vi "Start Daq.vi"(4 "AI voltage":dbl[](array[numeric]), 6 "AI Channels":string[](array[string]), 8 "error in":errorcluster, 9 "samples per read":i32=10 min=1 step=1, 10 "Data rate (hz)":dbl=500.0) -> (0 "error out":errorcluster, 3 "task out":refnum<k21>)   [LabVIEW 2015]
uses:
  <vilib>/DAQmx/create/channels.llb/DAQmx Create Channel (AI-Voltage-Basic).vi
  <vilib>/DAQmx/configure/timing.llb/DAQmx Timing (Sample Clock).vi
  <resource>/objmgr/daqmx.rc
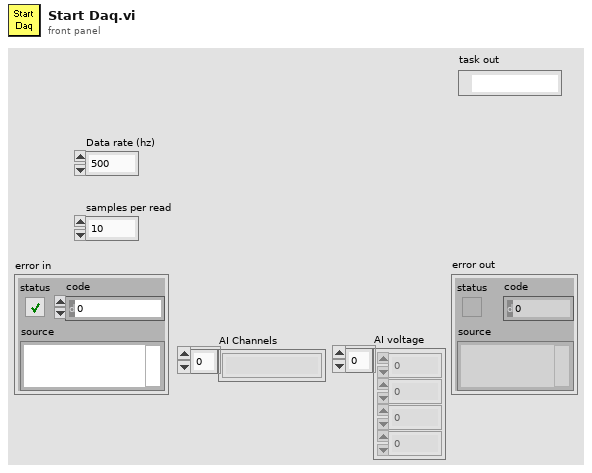
[diagram p1: front panel]
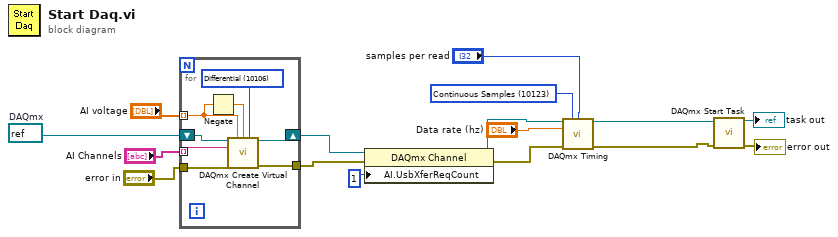
[diagram p0: block diagram]
diagram:
  w2 = refnum<k21> refnum  # DAQmx
  w9 = 10123 items=["Finite Samples"=10178, "Continuous Samples"=10123, "Hardware Timed Single Point"=12522] ("sample mode")
  n1 = for {
    tunnel: [w24] -> w15
    tunnel: "AI Channels" -> [w22] mode=indexing
    tunnel: "error in" -> [w21]
    shift-right: [w23] -> w14
    shift-left: w2 -> [w20]
    tunnel: "AI voltage" -> [w19] mode=indexing
    w17 = 10106 items=["default"=-1, "RSE"=10083, "NRSE"=10078, "Differential"=10106, "Pseudodifferential"=12529] ("input terminal configuration")
    n2 = Negate(x=w19) -> (-x=w18:dbl)
    n3 = call-poly <vilib>:"DAQmx Create Virtual Channel.vi"("task in"=w20, "maximum value"=w19, "minimum value"=w18, "input terminal configuration"=w17, "physical channels"=w22, "error in"=w21) -> ("task out"=w23:refnum<k21>, "error out"=w24:errorcluster)  [unwired: 8 in]
  }
  n4 = property class="DAQmx Channel"(reference=w14, error in=w15, "AI.UsbXferReqCount"=u32 1) -> (reference out=w11:refnum<k21>, error out=w12:errorcluster)
  n5 = call-poly <vilib>:"DAQmx Timing.vi"("task/channels in"=w11, "sample mode"=w9, "samples per channel"="samples per read", "rate"="Data rate (hz)", "error in"=w12) -> ("task out"=w8:refnum<k21>, "error out"=w7:errorcluster)  [unwired: 9 in]
  n6 = call <vilib>:"DAQmx Start Task.vi"("task/channels in"=w8, "error in"=w7) -> ("task out"=→"task out":refnum<k21>, "error out"=→"error out":errorcluster)  [unwired: 12 in]
